vi "GetTodayDateTime.vi"(11 "type":enum16{"StartTime", "EndTime"}(ring)) -> (3 "date":string)   [LabVIEW 2018]
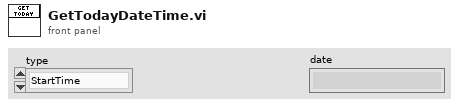
[diagram p1: front panel]
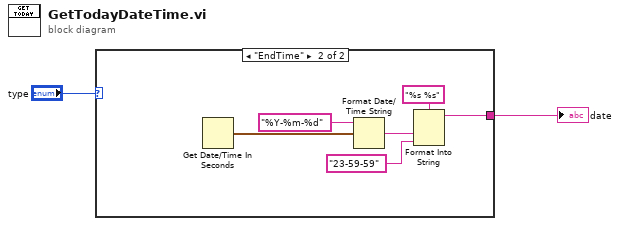
[diagram p0: block diagram]
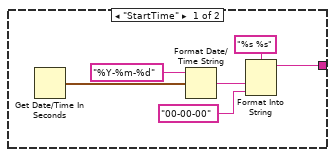
[diagram p2: hidden frame]
diagram:
  n1 = case shown="\"EndTime\"" "type" {
    tunnel: [w3 w9] -> w1
    frame "StartTime" {
      n2 = Get Date/Time In Seconds() -> (seconds since 1Jan1904=w7:timestamp)
      n3 = Format Date/Time String(time format string (%c)="%Y-%m-%d" ("시간 포맷 문자열 (%c)"), seconds (now)=w7) -> (date/time string=w5:string)  [unwired: 1 in]
      n4 = Format Into String(format string="%s %s" ("포맷 문자열"), w5, "00-00-00" ("입력 2")) -> (resulting string=w3:string)  [unwired: 2 in, 1 out]
    }
    frame "EndTime" {
      n5 = Get Date/Time In Seconds() -> (seconds since 1Jan1904=w13:timestamp)
      n6 = Format Date/Time String(time format string (%c)="%Y-%m-%d" ("시간 포맷 문자열 (%c)"), seconds (now)=w13) -> (date/time string=w11:string)  [unwired: 1 in]
      n7 = Format Into String(format string="%s %s" ("포맷 문자열"), w11, "23-59-59" ("입력 2")) -> (resulting string=w9:string)  [unwired: 2 in, 1 out]
    }
  }
  "date" <- w1
